vi "FdxAddIrigStructIrigCvi.vi"(8 "error in":errorcluster, 11 "IRIG IN A/B":T2) -> (0 "error out":errorcluster, 3 "IRIG OUT":T1)   [LabVIEW 2020, in "AIM664LV.lvlib"]
doc: "This function is used to calculate time tag sums. \nResult = IRIG Time A + IRIG Time B\n(Calculates with 366 Days / Year)"
uses:
  AIM664LV.lvlib
  AFDX_LibraryAdmin/FdxGlobalDllPath.vi
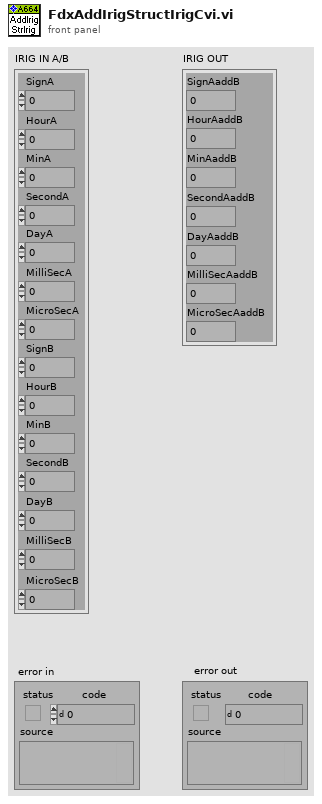
[diagram p1: front panel]
types:
  T1 = cluster{"SignAaddB":i32, "HourAaddB":u32, "MinAaddB":u32, "SecondAaddB":u32, "DayAaddB":u32, "MilliSecAaddB":u32, "MicroSecAaddB":u32}
  T2 = cluster{"SignA":i32, "HourA":u32, "MinA":u32, "SecondA":u32, "DayA":u32, "MilliSecA":u32, "MicroSecA":u32, "SignB":i32, "HourB":u32, "MinB":u32, "SecondB":u32, "DayB":u32, "MilliSecB":u32, "MicroSecB":u32}
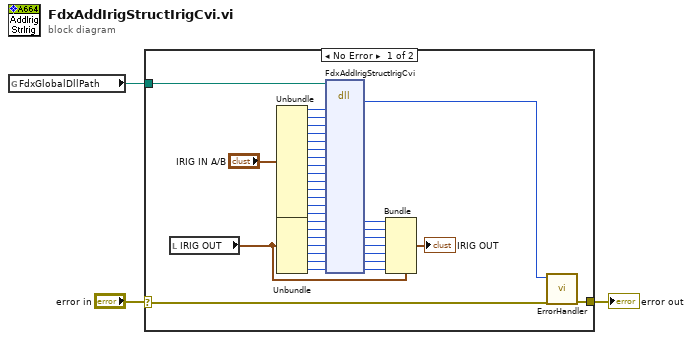
[diagram p0: block diagram]
diagram:
  n1 = global read "FdxGlobalDllPath.vi" "FdxGlobalDllPath"() -> (w1:path)
  n2 = case shown="No Error" "error in" {
    selector: "error in" -> [w37 w39]
    tunnel: [w38 w39] -> w3
    tunnel: w1 -> [w4 _]
    frame No Error {
      n3 = local read "IRIG OUT"() -> (w21:T1)
      n4 = Unbundle("IRIG IN A/B") -> ("SignA"=w33:i32, "HourA"=w32:u32, "MinA"=w31:u32, "SecondA"=w30:u32, "DayA"=w29:u32, "MilliSecA"=w28:u32, "MicroSecA"=w27:u32, "SignB"=w26:i32, "HourB"=w19:u32, "MinB"=w18:u32, "SecondB"=w17:u32, "DayB"=w16:u32, "MilliSecB"=w15:u32, "MicroSecB"=w14:u32)
      n5 = Unbundle(w21) -> ("SignAaddB"=w20:i32, "HourAaddB"=w10:u32, "MinAaddB"=w9:u32, "SecondAaddB"=w8:u32, "DayAaddB"=w7:u32, "MilliSecAaddB"=w6:u32, "MicroSecAaddB"=w5:u32)
      n6 = dll-call lib="aim_fdx.19.dll" fn="FdxAddIrigStructIrigCvi"(path in=w4, "SignA"=w33, "HourA"=w32, "MinA"=w31, "SecondA"=w30, "DayA"=w29, "MilliSecA"=w28, "MicroSecA"=w27, "SignB"=w26, "HourB"=w19, "MinB"=w18, "SecondB"=w17, "DayB"=w16, "MilliSecB"=w15, "MicroSecB"=w14, "SignAaddB"=w20, "HourAaddB"=w10, "MinAaddB"=w9, "SecondAaddB"=w8, "DayAaddB"=w7, "MilliSecAaddB"=w6, "MicroSecAaddB"=w5) -> ("status"=w36:i32, "SignAaddB"=w22:i32, "HourAaddB"=w23:u32, "MinAaddB"=w24:u32, "SecondAaddB"=w25:u32, "DayAaddB"=w13:u32, "MilliSecAaddB"=w12:u32, "MicroSecAaddB"=w11:u32)  [unwired: 16 in, 2 out]
      n7 = Bundle(cluster=w21, "SignAaddB"=w22, "HourAaddB"=w23, "MinAaddB"=w24, "SecondAaddB"=w25, "DayAaddB"=w13, "MilliSecAaddB"=w12, "MicroSecAaddB"=w11) -> (→"IRIG OUT":T1)
      n8 = call "ErrorHandler.vi"("error in"=w37, "AIM Error"=w36) -> ("error out"=w38:errorcluster)  [unwired: 9 in]
    }
    frame Error {
    }
  }
  "error out" <- w3
